vi "TC Range.vi"() -> ()   [LabVIEW 2020, in "Yokogawa GX Series.lvlib"]
uses:
  <instrlib>/Yokogawa GX Series/Yokogawa GX Series.lvlib
panel:
  in  "TC Range":string="R\nS\nB\nK\nK-H\nE\nJ\nT\nN\nW\nL\nU\nWRe3-25\nPLATINEL\nPR20-40\nKpvsAu7Fe\nNiNiMo\nWWRe26\nN14\nXK"
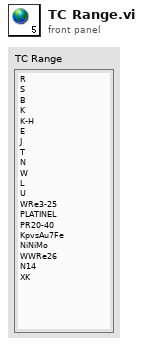
[diagram p1: front panel]
diagram:
